vi "LDF Exe Sch To Bus.vi"(9 "FillBitValue":u8, 10 "pSchName":string, 11 "LDFHandle":u64) -> (2 "pSchName out":string, 3 "function return":i32)   [LabVIEW 2010, in "ldf_parser.lvlib"]
doc: "int WINAPI LDF_ExeSchToBus(long long LDFHandle, char* pSchName, unsigned char FillBitValue);"
uses:
  ldf_parser.lvlib
  USB2XXX/trunk/USB2XXX/USB2XXX/vs2019/Release/USB2XXX.dll
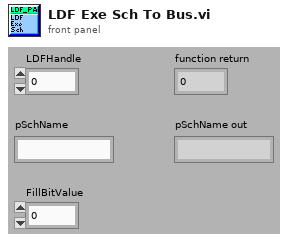
[diagram p1: front panel]
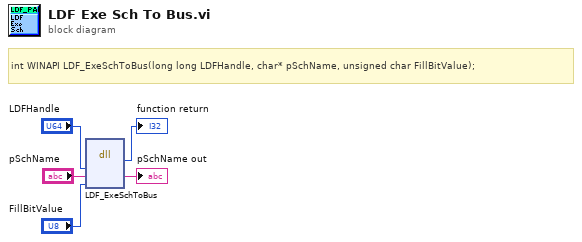
[diagram p0: block diagram]
diagram:
  # "int WINAPI LDF_ExeSchToBus(long long LDFHandle, char* pSchName, unsigned char FillBitValue);"
  n1 = dll-call lib="E:/Projects/USB2XXX/trunk/USB2XXX/USB2XXX/vs2019/Release/USB2XXX.*" fn="LDF_ExeSchToBus"("LDFHandle"="LDFHandle", "pSchName"="pSchName", "FillBitValue"="FillBitValue") -> (→"function return":i32, "pSchName"=→"pSchName out":string)  [unwired: 5 in, 2 out]
